vi "Summation Columns of Matrix.vi"(11 "A":T1) -> (3 "Summation Columns of A":dbl[](array[numeric]))   [LabVIEW 2020, in "NI_AALPro.lvlib"]
uses:
  <vilib>/Analysis/NI_AALPro.lvlib
  <vilib>/Analysis/Matrix/Datatypes/ComplexMatrix.ctl
  <vilib>/Analysis/Matrix/Numeric/Absolute Value/Absolute Value - CM.vi
  <vilib>/Analysis/Matrix/NI_Matrix.lvlib
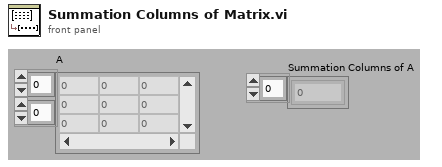
[diagram p1: front panel]
types:
  T1 = typedef "NI_Matrix.lvlib/ComplexMatrix.ctl" = cdb[][]
  T2 = typedef "NI_Matrix.lvlib/RealMatrix.ctl" = dbl[][]
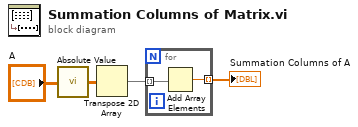
[diagram p0: block diagram]
diagram:
  n1 = call-poly <vilib>:"Absolute Value.vi"("Complex Matrix A"="A") -> ("|A|"=w3:T2)
  n2 = Transpose 2D Array(2D array=w3) -> (transposed array=w4:T2)
  n3 = for {
    tunnel: w4 -> [w6] mode=indexing
    tunnel: [w5] -> w1 mode=indexing
    n4 = Add Array Elements(numeric array=w6) -> (sum=w5:dbl)
  }
  "Summation Columns of A" <- w1
